vi "RemoveEntry.vi"(10 "Index":i32, 11 "Journal In":refnum<class "Journal.lvclass">) -> (3 "Journal Out":refnum<class "Journal.lvclass">)   [LabVIEW 2018, in "Journal.lvclass"]
uses:
  Journal.lvclass
  Journal.lvclass/Journal.ctl
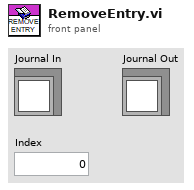
[diagram p1: front panel]
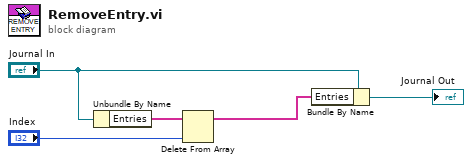
[diagram p0: block diagram]
diagram:
  n1 = Unbundle By Name("Journal In") -> ("Entries"=w3:string[])
  n2 = Delete From Array "Delete From Array"(array=w3, index="Index") -> (array with subset deleted=w2:string[])  [unwired: 1 in, 1 out]
  n3 = Bundle By Name(cluster="Journal In", "Entries"=w2) -> (→"Journal Out":refnum<class "Journal.lvclass">)
